vi "GlobalClicksHeight.vi"() -> ()   [LabVIEW 2017]
panel:
  in  "Zpos Graph (nm)":T1
  in  "Force, Current":cluster{"Current (pA)":dbl, "Fy (N)":dbl}
  in  "Frame properties (m)":cluster{cluster{dbl, dbl}, cluster{dbl, dbl}}
  in  "Position (nm)":cluster{"X":dbl, "Z":dbl, "Y":dbl}
  in  "Safe Tip?":bool
  in  "Starting Height (nm)":dbl
  out "Setpoint (A)":dbl=100.0
  out "Current (pA)":dbl
  in  "Found Surface?":bool
  out "Surface Location (nm)":dbl
  in  "Starting Height?":bool
  in  "Clicks and Height":bool
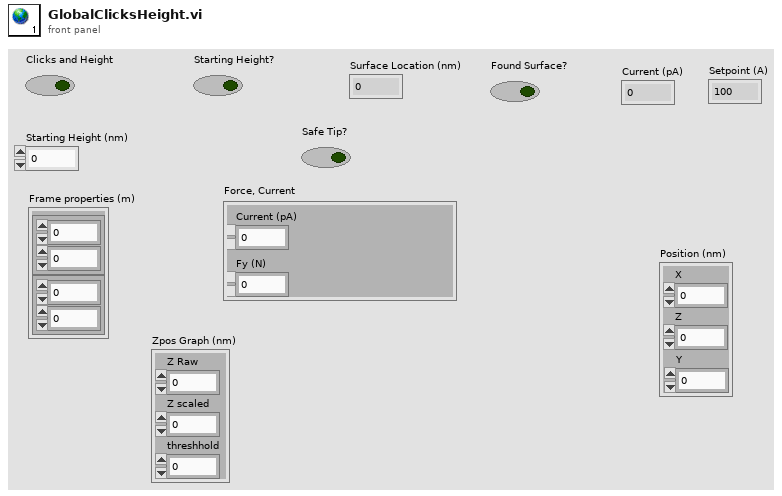
[diagram p1: front panel]
types:
  T1 = cluster{"Z Raw":dbl, "Z scaled":dbl, "threshhold":dbl}
diagram:
